vi "Execute.vi"(8 "error in":errorcluster, 11 "SUB in":refnum<class "SUB.lvclass">) -> (0 "error out":errorcluster, 1 "Next Step?":bool, 2 "MSG":string, 3 "SUB out":refnum<class "SUB.lvclass">)   [LabVIEW 2012, in "Sequence Composition.lvlib" / "SUB.lvclass"]
doc: "Pop the sequence stack and execute the resulting command on the sequence stack. If the command insists that we need to reinsert the current class, push it back onto the stack."
uses:
  SUB.lvclass
  STEPS/STEP.lvclass/STEP.ctl
  SEQ/SEQ.lvclass
  STEPS/STEP.lvclass
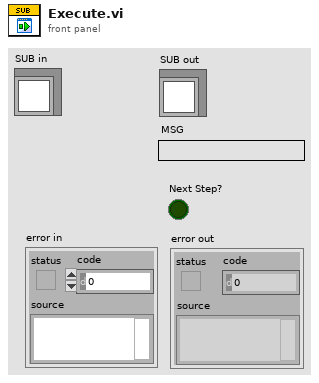
[diagram p1: front panel]
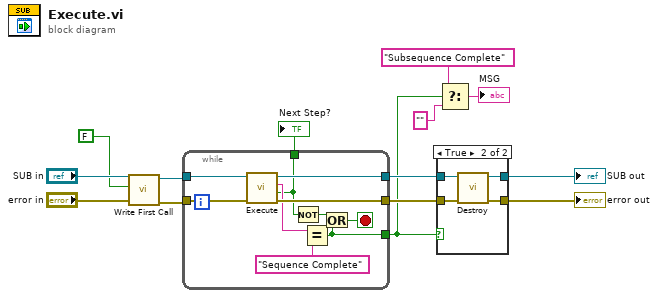
[diagram p0: block diagram]
diagram:
  n1 = call "Write First Call.vi"("error in"="error in", "First Call?"=FALSE, "STEP in"="SUB in") -> ("error out"=w1:errorcluster, "STEP out"=w2:refnum<class "SUB.lvclass">)  [unwired: 7 in]
  n2 = while {
    tunnel: w1 -> [w24]
    tunnel: w2 -> [w23]
    tunnel: [w17] -> w14
    tunnel: [w22] -> w13
    tunnel: [w21] -> w12
    tunnel: [w15] -> w7
    stop <- w16 stop-if-true
    n3 = call-parent "Execute.vi"("error in"=w24, "SEQ in"=w23) -> ("error out"=w21:errorcluster, "Next Step?"=w17:bool, "MSG"=w19:string, "SEQ out"=w22:refnum<class "SUB.lvclass">)  [unwired: 6 in]
    n4 = Not(x=w17) -> (.not. x?=w18:bool)
    n5 = Equal?(x=w19, y="Sequence Complete") -> (x = y?=w15:bool)
    n6 = Or(x=w18, y=w15) -> (x .or. y?=w16:bool)
  }
  "Next Step?" <- w14
  n7 = case shown="True" w7 {
    tunnel: w13 -> [w26 w30]
    tunnel: w12 -> [w25 w28]
    tunnel: [w26 w29] -> w10
    tunnel: [w25 w27] -> w11
    frame False {
    }
    frame True {
      n8 = call-dynamic "Destroy.vi"("error in"=w28, "SEQ in"=w30) -> ("error out"=w27:errorcluster, "SEQ out"=w29:refnum<class "SUB.lvclass">)  [unwired: 8 in]
    }
  }
  "error out" <- w11
  "SUB out" <- w10
  n9 = Select(t="Subsequence Complete", s=w7, f="") -> (s? t:f=→"MSG":string)
